vi "Nota de VF.vi"() -> ()   [LabVIEW 2016]
panel:
  in  "Nota de VC:":dbl format="%#.2f"
  in  "VE DE NÚMERO:":dbl[](array[numeric]) format="%#.2f"
  out "Nota de VF":dbl format="%#.2f"
  in  "Número de VEs":dbl format="%#14.2f"
  # "CÁLCULO DA NOTA DE VF"
  # "1) Dígite o Número de VEs:"
  # "2) Dígite as Notas de VEs:"
  # "3) Dígite as Nota de VC:"
  # "4) RODE O PROGRAMA :"
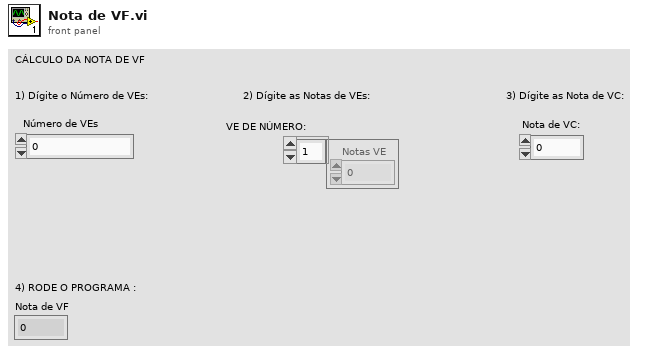
[diagram p1: front panel]
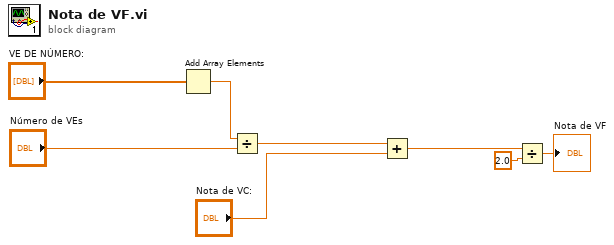
[diagram p0: block diagram]
diagram:
  n1 = Add Array Elements(numeric array="VE DE NÚMERO:") -> (sum=w1:dbl)
  n2 = Divide(x=w1, y="Número de VEs") -> (x/y=w8:dbl)
  n3 = Add(x=w8, y="Nota de VC:") -> (x+y=w6:dbl)
  n4 = Divide(x=w6, y=2.0 ("VC 2")) -> (x/y=→"Nota de VF":dbl)
